vi "Flow_path_prediction.vi"() -> ()   [LabVIEW 2013]
panel:
  out "error IO":errorcluster
  in  "error constant":errorcluster
  out "path predictor":picture
  in  "v":dbl(slide) scale=-3.0..3.0
  in  "u":dbl(slide) scale=-3.0..3.0
  in  "stop":bool
  # "meter/seconds"
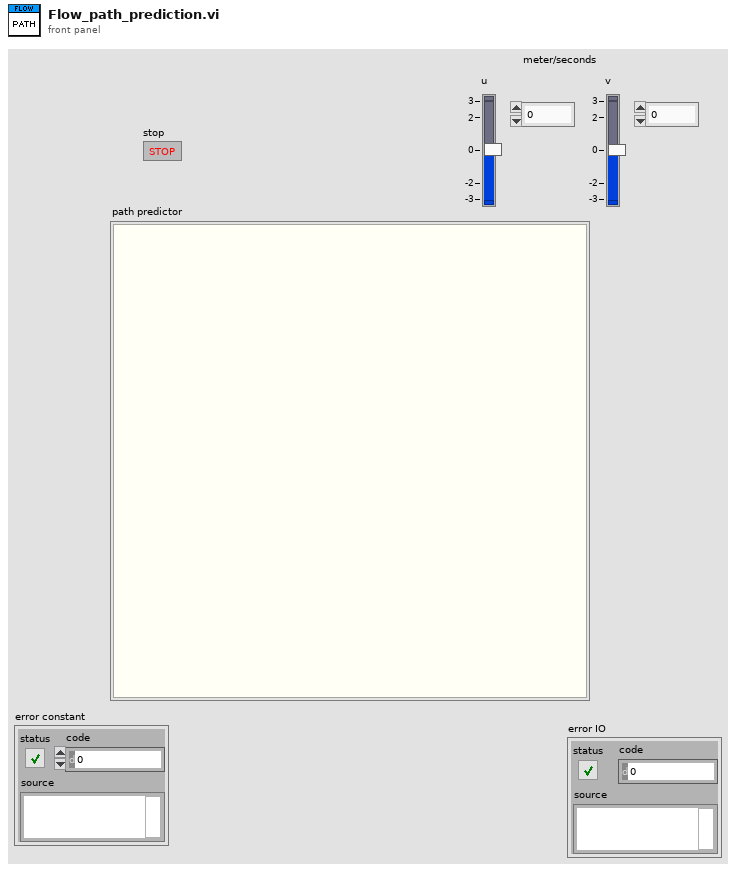
[diagram p1: front panel]
types:
  T1 = cluster{"Width":u16, "Style":enum32{"Solid", "Dash", "Dot", "DashDot", "DashDotDot"}}
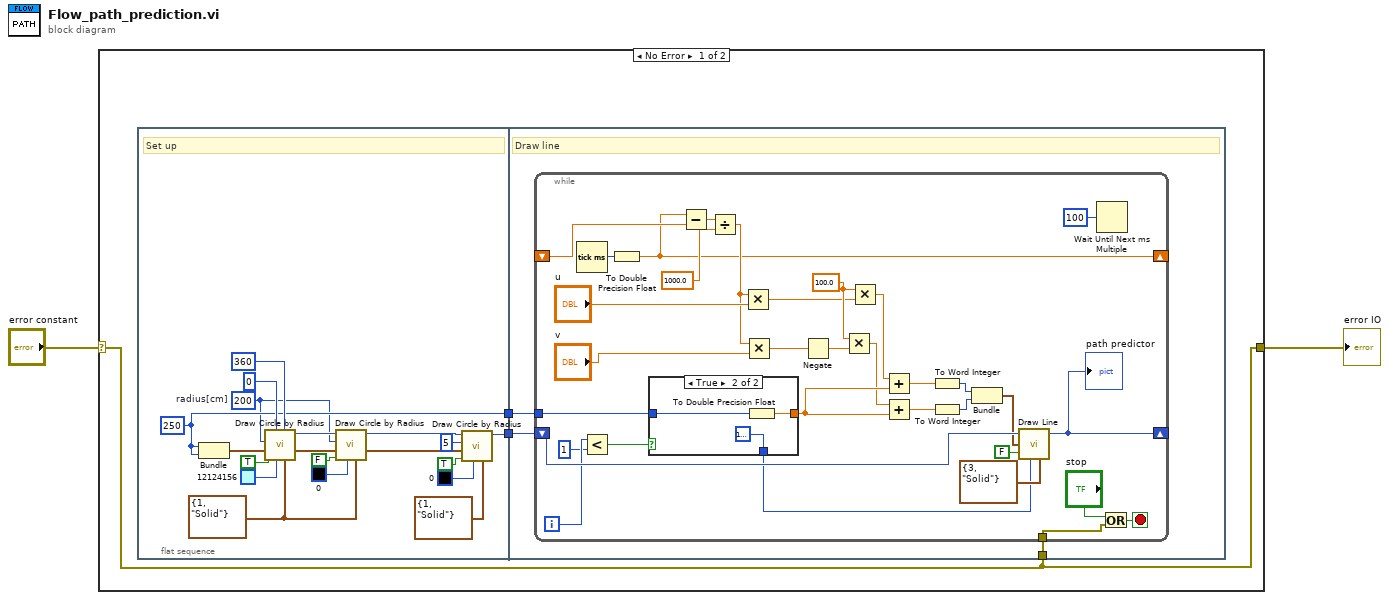
[diagram p0: block diagram]
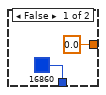
[diagram p2: hidden frame]
diagram:
  n1 = case shown="No Error" "error constant" {
    selector: "error constant" -> [w3 w64]
    tunnel: [w3 w64] -> w1
    frame No Error {
      n2 = flat-sequence {
        tunnel: [w17] -> w5
        tunnel: [w19] -> w4
        tunnel: w5 -> [w25]
        tunnel: w4 -> [w24]
        tunnel: w3 -> [w23]
        frame #0 {
          w19 = i16 250 ("horizontal")
          w7 = T1 {"Width"=1, "Style"=enum."Solid"} ("pen")
          w6 = i16 200  # radius[cm]
          # "Set up"
          n3 = Bundle("horizontal"=w19, "horizontal"=w19) -> (w10:cluster{"horizontal":i16, "horizontal":i16})  [unwired: 1 in]
          n4 = call <vilib>:"Draw Circle by Radius.vi"("pen"=w7, "arc size(360)"=i16 360, "color(black)"=u32 12124156, "start angle(0)"=i16 0, "fill?(F)"=TRUE, "pixel center"=w10, "radius"=w6) -> ("new picture"=w12:picture)  [unwired: 4 in]
          n5 = call <vilib>:"Draw Circle by Radius.vi"("pen"=w7, "color(black)"=u32 0, "fill?(F)"=FALSE, "pixel center"=w10, "radius"=w6, "picture"=w12) -> ("new picture"=w11:picture)  [unwired: 5 in]
          n6 = call <vilib>:"Draw Circle by Radius.vi"("pen"=T1 {"Width"=1, "Style"=enum."Solid"}, "color(black)"=u32 0, "fill?(F)"=TRUE, "pixel center"=w10, "radius"=i16 5, "picture"=w11) -> ("new picture"=w17:picture)  [unwired: 5 in]
        }
        frame #1 {
          # "Draw line"
          n7 = while {
            shift-right: [w47] -> _
            shift-left: _ -> [w48]
            shift-right: [w51] -> _
            shift-left: w25 -> [w52]
            tunnel: w24 -> [w44]
            tunnel: w23 -> [w27]
            i -> [w43]
            stop <- w28 stop-if-true
            w37 = 100.0 ("x")
            n8 = Tick Count (ms)() -> (millisecond timer value=w58:u32)
            n9 = Less?(x=w43, y=1) -> (x < y?=w29:bool)
            n10 = To Double Precision Float(number=w58) -> (double precision float=w47:dbl)
            n11 = case shown="True" w29 {
              tunnel: [0.0 w62] -> w45
              tunnel: w44 -> [_ w61]
              tunnel: [u32 16860 ("color(black)") u32 16777216 ("color(black)")] -> w41
              frame False {
              }
              frame True {
                n12 = To Double Precision Float(number=w61) -> (double precision float=w62:dbl)
              }
            }
            n13 = Subtract(x=w47, y=w48) -> (x-y=w55:dbl)
            n14 = Divide(x=w55, y=1000.0) -> (x/y=w54:dbl)
            n15 = Multiply(x=w54, y="u") -> (x*y=w36:dbl)
            n16 = Multiply(x=w54, y="v") -> (x*y=w35:dbl)
            n17 = Negate(x=w35) -> (-x=w38:dbl)
            n18 = Multiply(x=w37, y=w38) -> (x*y=w39:dbl)
            n19 = Multiply(x=w37, y=w36) -> (x*y=w40:dbl)
            n20 = Add(x=w40, y=w45) -> (x+y=w34:dbl)
            n21 = Add(x=w39, y=w45) -> (x+y=w32:dbl)
            n22 = To Word Integer(number=w34) -> (16bit integer=w33:i16)
            n23 = To Word Integer(number=w32) -> (16bit integer=w31:i16)
            n24 = Bundle(w33, w31) -> (w46:cluster{i16, i16})  [unwired: 1 in]
            n25 = call <vilib>:"Draw Line.vi"("picture"=w52, "end point"=w46, "absolute coordinates?(T)"=FALSE, "color(black)"=w41, "pen"=T1 {"Width"=3, "Style"=enum."Solid"}) -> ("new picture"=w51:picture)  [unwired: 4 in]
            "path predictor" <- w51
            n26 = Wait Until Next ms Multiple(millisecond multiple=u32 100) -> ()  [unwired: 1 out]
            n27 = Or(x="stop", y=w27) -> (x .or. y?=w28:bool)
          }
        }
      }
    }
    frame Error {
    }
  }
  "error IO" <- w1
